vi "0~10v 250bar.vi"(1 "Voltage V":dbl) -> (0 "Pressure bar":dbl)   [LabVIEW 2024]
doc: "Scale the 0-10V to 0-250 bar range."
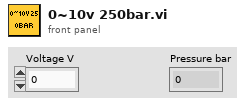
[diagram p1: front panel]
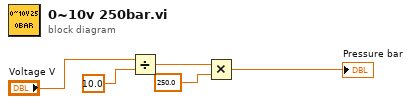
[diagram p0: block diagram]
diagram:
  n1 = Divide(x="Voltage V", y=10.0) -> (x/y=w3:dbl)
  n2 = Multiply(x=w3, y=250.0) -> (x*y=→"Pressure bar":dbl)
